vi "Save Multirate Filter to Text File.vi"() -> ()   [LabVIEW 2023]
doc: "Demonstrates how to use the DFD Save MRate to Text File VI to export a multirate filter into a text file.\n\nComplete the following steps to use this VI.\n1) Configure the <B>Quantize the Multirate Filter?</B> option. If you want to quantize the floating-point multirate filter to a fixed-point multirate filter, set this input to TRUE. Otherwise, set this input to FALSE. \n2) Run the VI.\n3) On the dialog box that appears, specify the path to the file in which you want to save the multirate filter and click the <B>OK</B> button."
uses:
  <vilib>/addons/Digital Filter Design/Design.llb/DFD MRate Filter Design (Integer).vi
  <vilib>/addons/Digital Filter Design/FilterLib.llb/DFD Save MRate Filter to Text File.vi
  <vilib>/addons/Digital Filter Design/NI_DigFilterLicensed.lvlib
panel:
  out "Error Message":string
  out "Text":string
  out "Target File Path":path
  in  "Quantize the Multirate Filter?":bool
  # "Select Help>>Show Context Help and move the cursor over the VI icon for more information."
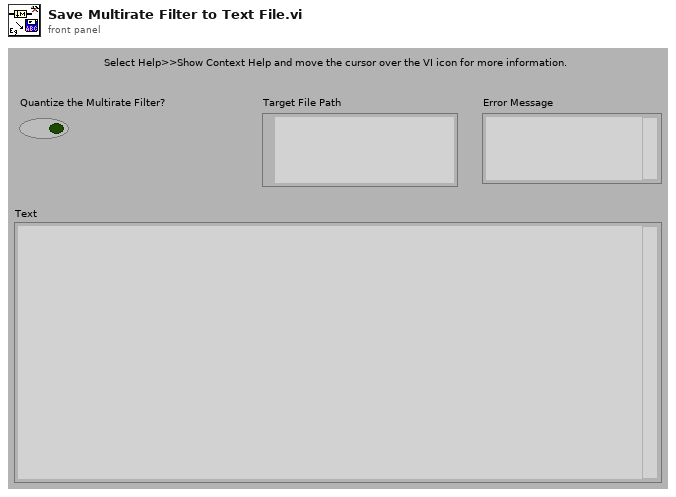
[diagram p1: front panel]
types:
  T1 = typedef "NI_DigFilterLicensed.lvlib/DFD Multirate Filter Obj.ctl" = cluster{"mMRate_Structure":enum16{"CIC", "FIR", "IIR", "Lattice"}, "mMRate_Mode":T2, "mMRate_Factor":i32, "mMRate_FIRParams":cluster{"mMRate_FIR_H":dbl[], "mMRate_FIR_IsNyquist?":bool, "mMRate_FIR_IsSymmetric?":bool}, "mMRate_CICParams":cluster{"mMRate_CIC_#Stage":i32, "mMRate_CIC_Lag":i32, "mMRate_CIC_Type":enum16{"Lowpass", "Highpass"}}, "mMRate_Order":i32, "mMRate_Version":string, "mMRate_Comments":string, "mMRate_RationalFactor":cluster{"mMRate_L":i32, "mMRate_M":i32}, "mMRate_Fs":dbl, "mMRate_Quantized?":bool, "mMRate_QFilterGain":dbl, "mMRate_CoefWl":i16, "mMRate_Scaling":cluster{"mMRate_ScaleByPowerOf2?":bool, "mMRate_ScaleType":T3}, "mMRate_InputWl":i16, "mMRate_OutputWl":i16, "mMRate_OutputMode":T4, "mMRate_MultMode":T5, "mMRate_BitPruning":bool, "mMRate_GainWl":i16, "mMRate_OutputFwl":i16, "mMRate_SumIwl":i16, "mMRate_InputIwl ":i16, "mMRate_SumWl":i16, "mMRate_CoefIwl":i16}
  T2 = typedef "NI_DigFilterLicensed.lvlib/DFD Multirate Mode.ctl" = i16
  T3 = typedef "NI_DigFilterLicensed.lvlib/DFD Coef Norm Type.ctl" = enum16{"No Norm", "Time Domain 1-Norm", "Time Domain 2-Norm", "Time Domain Inf-Norm"}
  T4 = typedef "NI_DigFilterLicensed.lvlib/DFD Round-off Mode.ctl" = enum16{"Nearest", "Truncation"}
  T5 = typedef "NI_DigFilterLicensed.lvlib/DFD FXP MRate Multiply Mode.ctl" = enum16{"Truncated", "Full"}
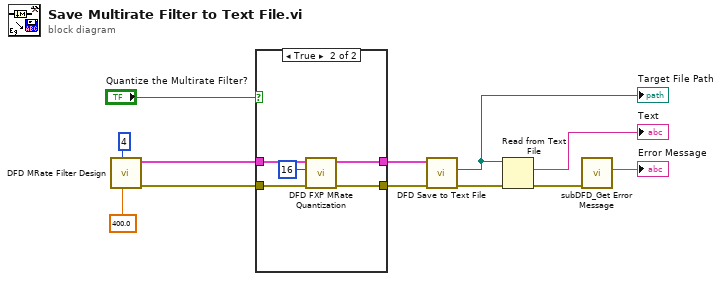
[diagram p0: block diagram]
diagram:
  n1 = call-poly <vilib>:"DFD MRate Filter Design.vi"("fs in [Hz]"=400.0, "factor"=4) -> ("error out"=w5:errorcluster, "multirate filter out"=w10:T1)  [unwired: 6 in, 2 out]
  n2 = case shown="True" "Quantize the Multirate Filter?" {
    tunnel: w10 -> [w14 w19]
    tunnel: [w14 w17] -> w8
    tunnel: w5 -> [w13 w16]
    tunnel: [w13 w15] -> w4
    frame False {
    }
    frame True {
      n3 = call <vilib>:"DFD FXP MRate Quantization.vi"("error in (no error)"=w16, "coefficients word length"=i16 16 ("coefficients wl"), "multirate filter in"=w19) -> ("error out"=w15:errorcluster, "multirate filter out"=w17:T1)  [unwired: 3 in, 4 out]
    }
  }
  n4 = call-poly <vilib>:"DFD Save to Text File.vi"("error in (no error)"=w4, "multirate filter in"=w8) -> ("error out"=w3:errorcluster, "file path out"=w7:path)  [unwired: 2 in, 6 out]
  "Target File Path" <- w7
  n5 = Read from Text File(file (use dialog)=w7, error in=w3) -> (text=→"Text":string, error out=w2:errorcluster)  [unwired: 4 out]
  n6 = call <vilib>:"subDFD_Get Error Message.vi"("error in (no error)"=w2) -> ("Error Message"=→"Error Message":string)  [unwired: 10 out]
